vi "02 HEWH Heat Up Test SM1.vi"(0 "Equipment":T6={"MW100"="COM3", "AG34970"="MW100", "WT210"="A-34972A"}, 5 "Degree Setting":dbl=58.0, 7 "Flow rate setting":dbl=3.0, 11 "Error In":errorcluster) -> (15 "Error Out":errorcluster)   [LabVIEW 2014]
uses:
  <vilib>/Utility/file.llb/Write To Spreadsheet File (string).vi
  Type Definitions/Use Modes.ctl
  Type Definitions/HEWH_Mode.ctl
  Type Definitions/ValveBankPositions.ctl
  Type Definitions/Intellfaucet Mode.ctl
  <vilib>/Analysis/NI_AALBase.lvlib
  <vilib>/Analysis/baseanly.llb/Mean (DBL).vi
  Type Definitions/EquipReferences.ctl
  Type Definitions/Heating Modes.ctl
  Type Definitions/HEWH Tank Indicator.ctl
  Type Definitions/PowerElements.ctl
  Type Definitions/TestedFlowratesScenarios.ctl
panel:
  in  "Test Condition":T1=enum."Global, Tank"
  out "Label Array":string[](array[string])
  out "Use Agilent?":bool
  out "Voltage":dbl=240.0
  out "COM Port":refnum<visa-resource-name>
  out "Serial Data In":string
  out "LAN IP Address":string="192.168.25.3"
  out "Computer Name":string
  out "Ver.":string
  out "POWER":T2
  out "Tank Display":T3 {"TC6" format="%.2g"; "TIN" format="%.2g"; "TOUT" format="%.2g"; "Mean" format="%.2f"; "Std Dev" format="%.2f"; "TC5" format="%.2g"; "TC4" format="%.2g"; "TC3" format="%.2g"; "TC2" format="%.2g"; "TC1" format="%.2g"}
  in  "Function Tab":enum32{"Setup", "Test Status", "Charts"}(tab)
  out "MW100":refnum<visa-resource-name>
  out "FileName":path
  in  "Working File Directory":path=path "c:/data"
  out "Heating  Mode":T4=enum."Hybrid Heating"
  in  "DRM Mode":T5=3 items=["CRITICAL", "HIGH", "MEDIUM", "Normal"]
  out "Data Array":string[][](array[string])
  out "GEA2 HyperData":bool=TRUE
  in  "Expansion Tank?":bool=TRUE
  in  "Status Tab":T7(tab)=enum."Feedback 6"
  out "errorset mode":errorcluster
  out "Init Complete":bool
  out "Mode":T8=enum."HighDemand"
  out "Set Point":u8=140
  out "Heat Source Indicator":bool
  in  "SkipStabilize":bool
  out "Elapsed Time (secs)":dbl format="%.2f"
  in  "Stability Sample Delay(s)":dbl=120.0
  out "1.Delay Mins(30)":dbl
  in  "1.SkipDelay":bool
  out "Flowrate adj":dbl=3.0
  out "Downspout Flow Chart":dbl(graph)=3.8899999999999997
  in  "Time Delay(30)":dbl=30.0
  out "Temp adj":dbl=3.0
  out "Downspout Temp":dbl(graph)=3.8899999999999997
  out "2.Bottom Source Indicator":bool
  in  "2. Initial Draw":dbl=10.75
  out "3.WaitTime(10min)":dbl
  out "error 3":errorcluster
  out "3.Heat Source Indicator":bool
  in  "Wait Time(600s)":dbl=600.0
  out "4.Delay Remaining (300s)":dbl
  in  "Delay(300s)":dbl=300.0
  in  "4.Skip Delay":bool
  out "Downspout Flow Chart":dbl(graph)=3.8899999999999997
  out "Downspout Flow":dbl=3.8899999999999997
  out "Total Gal Out":dbl
  out "5.Top Source Indicator":bool
  in  "Eheat Gal Limit":dbl=40.0
  in  "Flow Adjust Time (3s)":dbl=1.5
  in  "K(0.1)":dbl=0.1
  in  "Total Gal Limit":dbl=200.0
  out "6.Bottom Source Indicator":bool
  in  "Delay eHeat Command (mS)":u32=15000
  in  "Skip Waiting for Bottom Source to turn off.":bool
  out "7.Heat Source Indicator":bool
  out "Mean Tank Temp":dbl
  in  "Min Ave Temp Limit":dbl=120.0
  in  "8.Skip Waiting":bool
  out "Seconds to Completion":dbl
  in  "8.Delay(1800s)":dbl=1800.0
  out "LoggingStopped":bool=TRUE
  out "Test Data":string[][](array[string])
  in  "Graph Tab":enum32{"Temperature", "Power", "Gallons"}(tab)
  out "Ave Temp":dbl format="%0.2f"
  out "Local?":bool
  # "Select the Modes for the test.  This will need to be\nset up on the water heater."
  # "Wait for stabilization.  Checks heat sources every second.  \nIf the heat sources are both off, the water heater is stabilized. \nFor StdElect. Looks at the heating element.  For other heating\nmodes, looks at the RS232 feedback on fans and compressor."
  # "\"1.\tAfter unit has been stable for 30+/-5 minutes, Open valve,\n and draw 10.75 +/- .25 gallons of water at a rate of 3+/-.25 gpm.\""
  # "First, Allow the water temp and flow to stabilize in the downspout,\nthen switch to the tank."
  # "\"2.\tIf lower heat source energizes (Hybrid Mode/eHeat Mode = FAN ON\nfollow by Compressor, Standard Electric Mode = Lower Element ON) \nbefore 10.75 gallons, then continue drawing water until Upper element \nengages as shown in step 5 (skip to step 5).\""
  # "\"3.\tIf lower heat source does not energize during 10.75 gallon draw, then wait a maximum of 10 minutes to see if lower heat source will energize.  If it does, then\nallow the water heater to recover to set point.\""
  # "\"4.\tAllow unit to sit 5 to 10 minutes in stabilized conditions, then:\""
  # "Change delay value to skip ahead."
  # "\"5.\tOpen valve and draw water at 3+/-.25 gpm until the Upper Element \nenergizes.  Water draw must stop within 5 seconds after Upper Element \nenergizes.  NOTE: when running the unit in e-Heat mode, (no upper \nelement) draw 40+/-0.25 gallons of water.\""
  # "\"6.\tIn Hybrid Mode: when the Upper Element stops and \nswitches to Lower Element, switch the unit to eHeat Mode.  \nThis will switch the lower heating source to Compressor.\""
  # "Since there may be a significant delay \nfor the compressor to turn on, also check \nto make sure that the mean tank temp\nis above some limit."
  # "7.\tAllow water heater to stabilize this second time. \n(Recover water temperature back to set point)."
  # "8.\tAllow unit to sit a minimum of 30 minutes in stabilized conditions, then;"
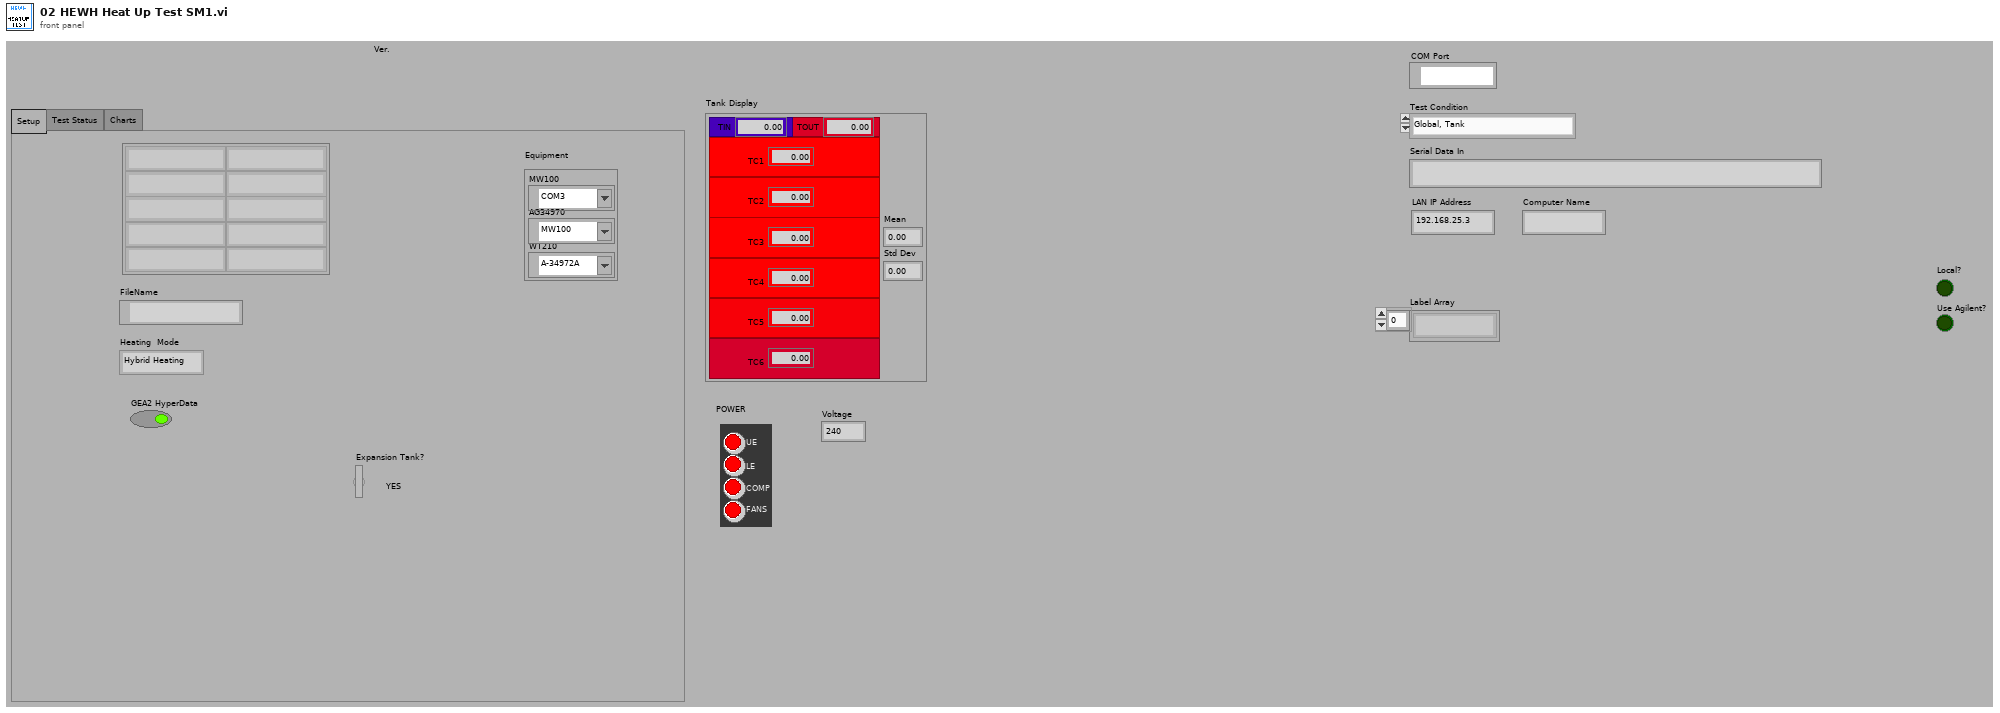
[diagram p1: front panel]
types:
  T1 = typedef "TestedFlowratesScenarios.ctl" = enum16{"DRK500,Station1", "DRK375,Lab", "SRK500,Station1,5GPM FR", "DRK375,STATION3,1/2\"HOSE", "DRK500,Station1,downspout", "DRK375,Station3,thruEcocute", "DRK375,Station3,purge", "Build2,2B,Purge", "Global, Purge", "Global, Tank", "DRK250"}
  T2 = typedef "PowerElements.ctl" = cluster{"UE":bool, "LE":bool, "COMP":bool, "FANS":bool}
  T3 = typedef "HEWH Tank Indicator.ctl" = cluster{"TC1-D":bool, "TC2-D":bool, "TC3-D":bool, "TC4-D":bool, "TC5-D":bool, "RTD_IN":bool, "RTDOUT":bool, "TC1":dbl, "TC2":dbl, "TC3":dbl, "TC4":dbl, "TC5":dbl, "TIN":dbl, "TOUT":dbl, "Std Dev":dbl, "Mean":dbl, "TC6-D":bool, "TC6":dbl}
  T4 = typedef "Heating Modes.ctl" = enum16{"Standard Electric", "Hybrid Heating", "E-Heat Mode"}
  T5 = typedef "Use Modes.ctl" = u16
  T6 = typedef "EquipReferences.ctl" = cluster{"MW100":refnum<visa-resource-name>, "AG34970":refnum<visa-resource-name>, "WT210":refnum<visa-resource-name>}
  T7 = enum32{"External Program Controls", "External Program Controls 2", "Program Controls", "Feedback", "Feedback 2", "Feedback 3", "Feedback 4", "Feedback 5", "Feedback 6", "Feedback 7", "Feedback 8", "Feedback 9", "Feedback 10"}
  T8 = typedef "HEWH_Mode.ctl" = enum16{"Hybrid", "StdElectric", "eHeat", "HighDemand", "Vacation"}
  T9 = typedef "Intellfaucet Mode.ctl" = enum16{"Adjust Temp", "Adjust Flow", "Start Flow", "Stop Flow"}
  T10 = typedef "ValveBankPositions.ctl" = enum16{"Heating", "Purge", "Resting", "Draw"}
  T11 = typedef "FileVersionInformation.ctl" = cluster{"FileVersion":string, "ProductName":string, "InternalName":string, "CompanyName":string, "LegalCopyright":string, "FileDescription":string}
  T12 = enum16{"Computation Start", "Computation stop", "Reset Computation", "Clear Computation"}[]
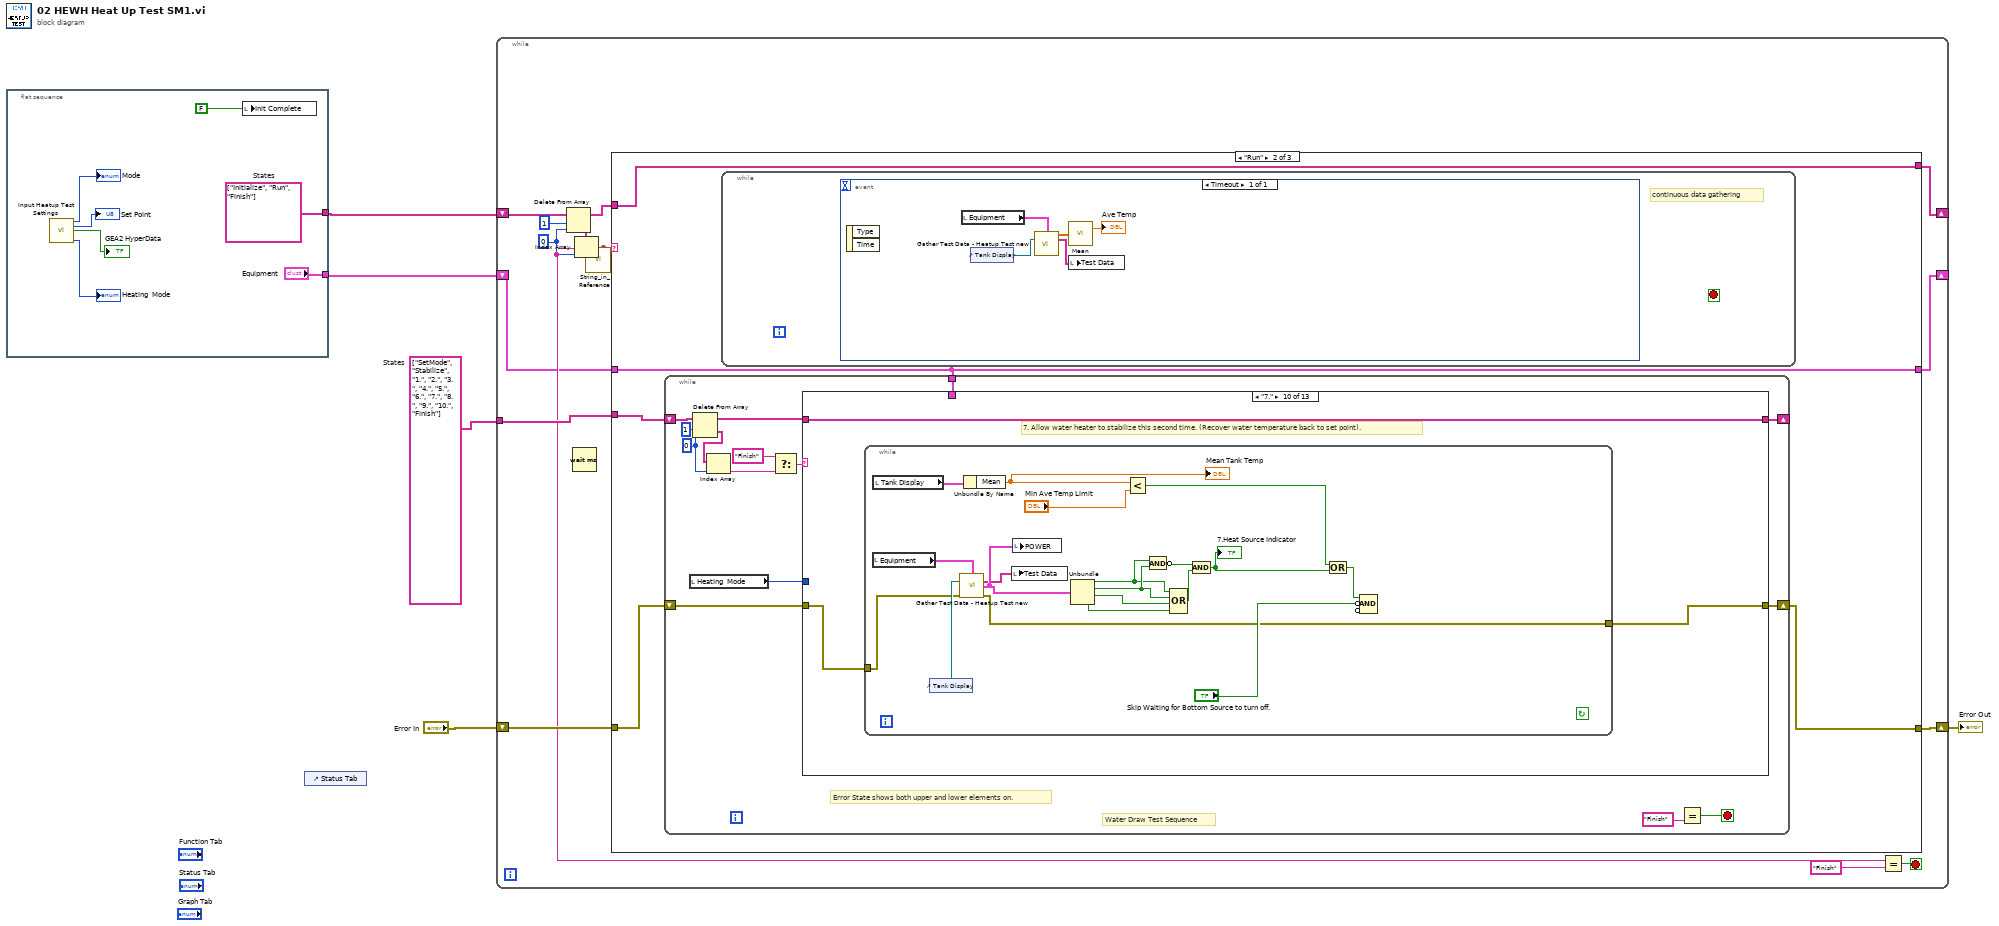
[diagram p0: block diagram]
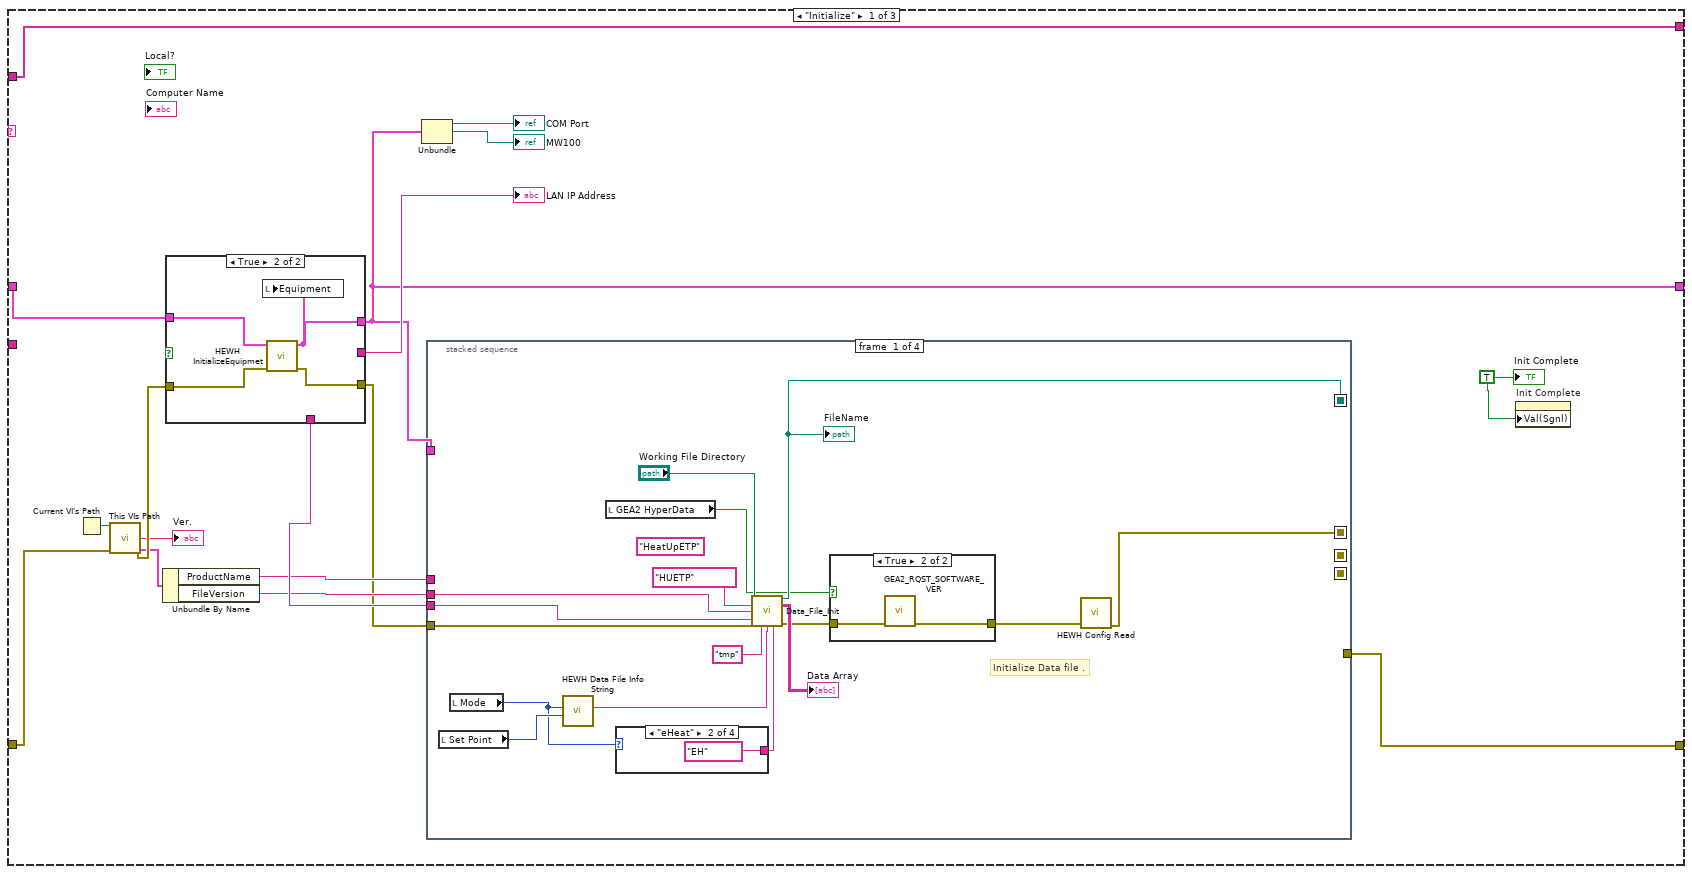
[diagram p2: hidden frame]
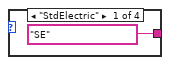
[diagram p4: hidden frame]
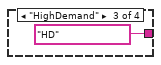
[diagram p5: hidden frame]
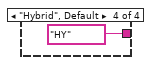
[diagram p6: hidden frame]
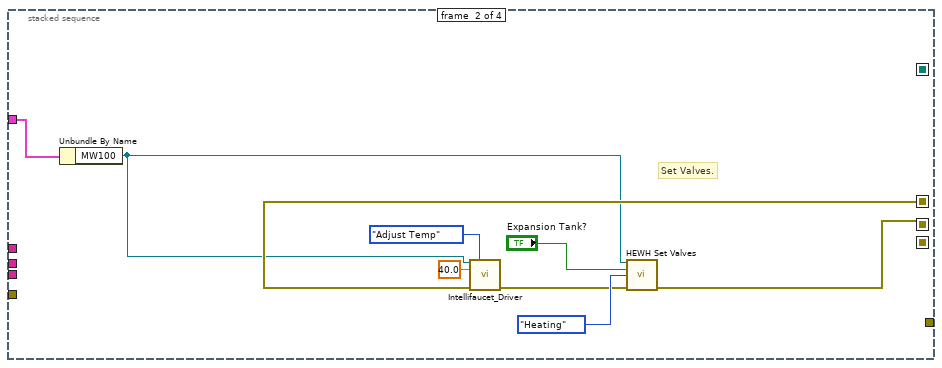
[diagram p7: hidden frame]
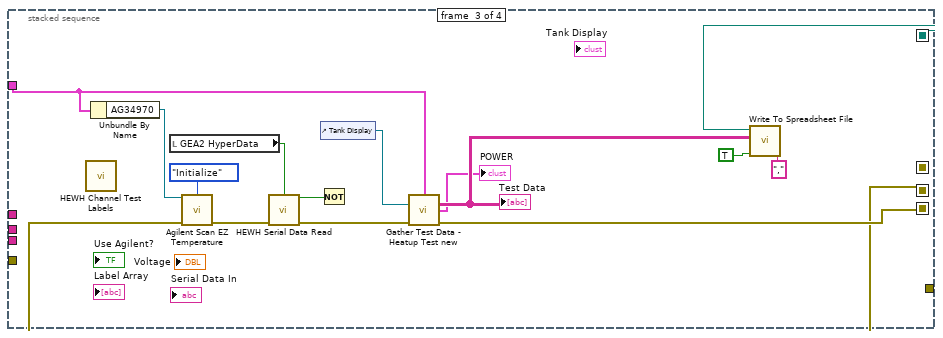
[diagram p8: hidden frame]
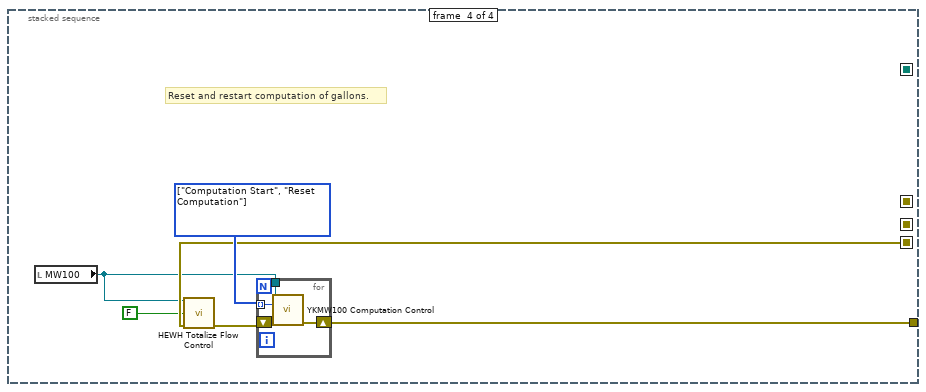
[diagram p9: hidden frame]
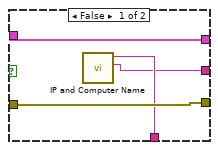
[diagram p10: hidden frame]
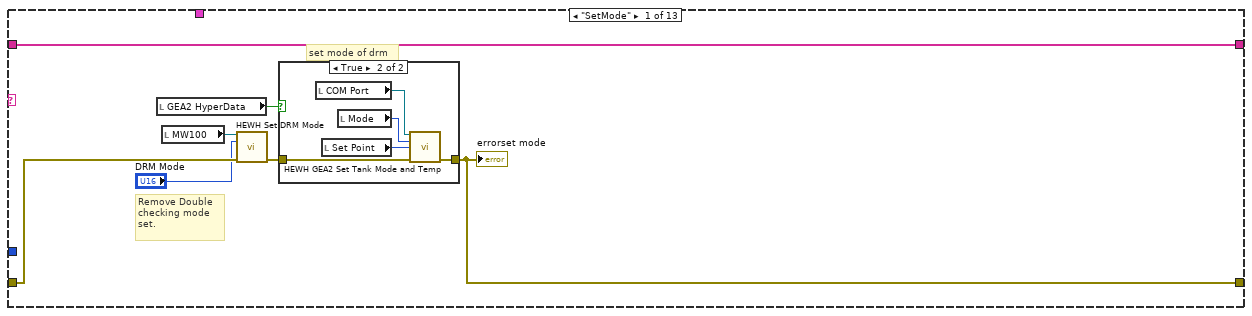
[diagram p11: hidden frame]
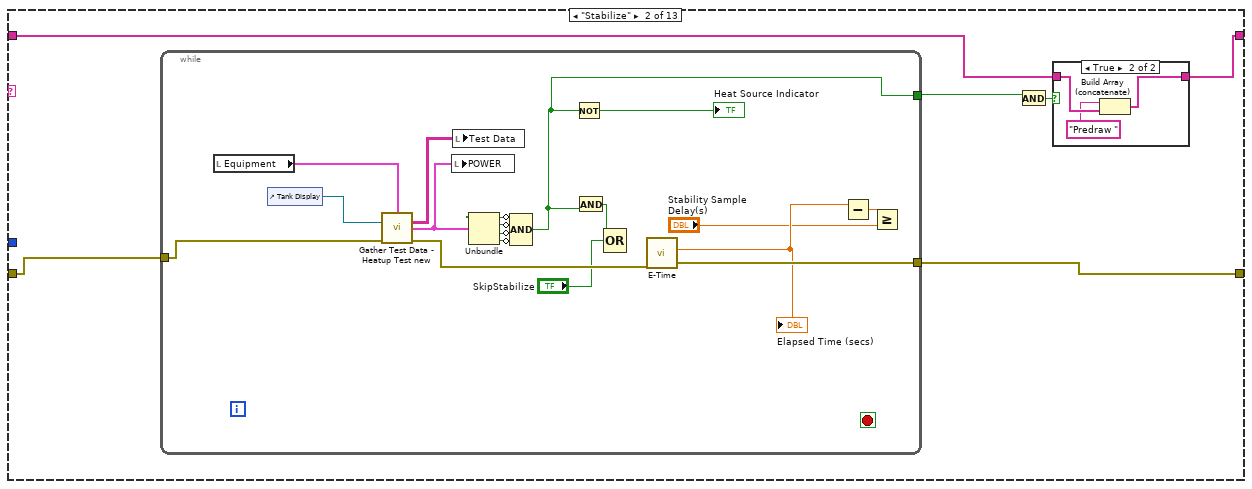
[diagram p13: hidden frame]
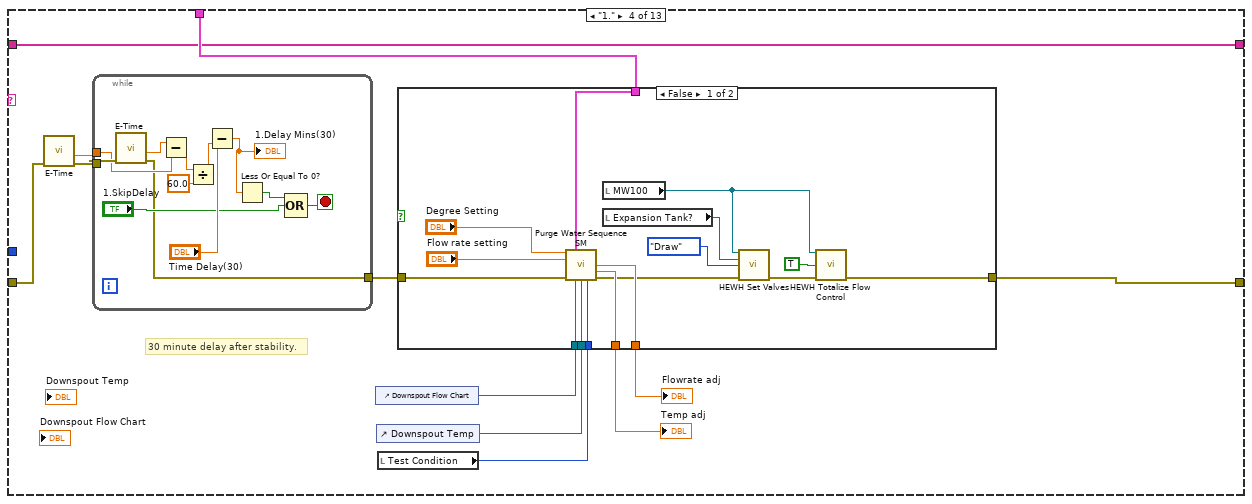
[diagram p16: hidden frame]
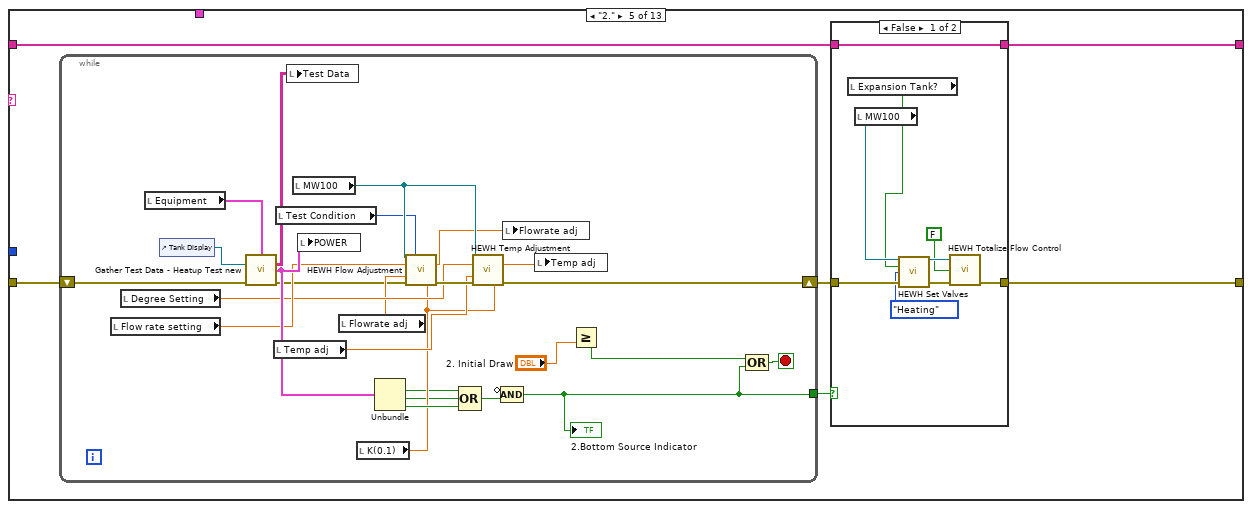
[diagram p18: hidden frame]
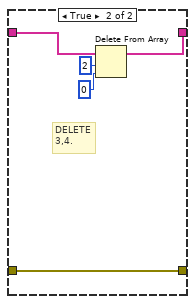
[diagram p19: hidden frame]
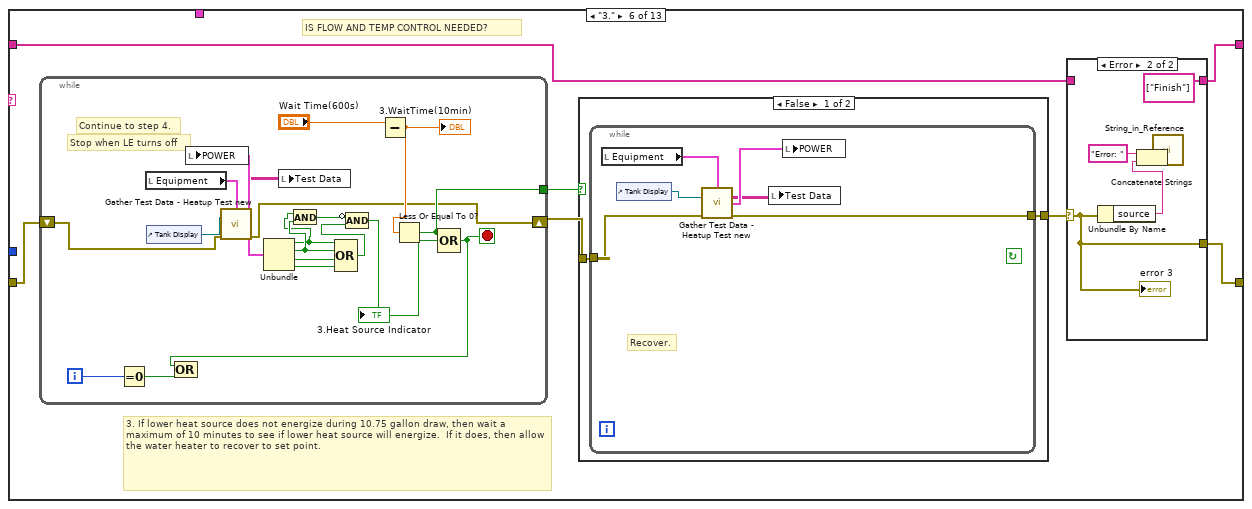
[diagram p20: hidden frame]
diagram:
  w3 = string[] ["SetMode", "Stabilize", "1.", "2.", "3.", "4.", "5.", "6.", "7.", "8.", "9.", "10.", "Finish"]  # States
  n1 = flat-sequence {
    tunnel: [w12] -> w5
    tunnel: ["Equipment"] -> w1
    frame #0 {
      w12 = string[] ["Initialize", "Run", "Finish"]  # States
      n2 = call "Input Heatup Test Settings.vi"() -> ("GEA2 Set Mode Out"=→"Mode":T8, "Set PointOut"=→"Set Point":u8, "GEA2 HyperData Out"=→"GEA2 HyperData":bool, "Heating  Mode Out"=→"Heating  Mode":T4)  [unwired: 11 in, 1 out]
      n3 = local write "Init Complete"(FALSE ("Init Complete")) -> ()
    }
  }
  n4 = control-ref of="Status Tab"() -> ()  [unwired: 1 out]
  n5 = while {
    shift-right: [w22] -> _
    shift-left: w5 -> [w26]
    shift-right: [w20] -> w4
    shift-left: "Error In" -> [w19]
    shift-right: [w16] -> _
    shift-left: w1 -> [w13]
    tunnel: w3 -> [w15]
    stop <- w18 stop-if-true
    w23 = 0 ("index")
    n6 = Delete From Array(array=w26, length=1, index=w23) -> (deleted portion=w24:string[], array with subset deleted=w21:string[])
    n7 = Wait (ms)() -> ()  [unwired: 1 in, 1 out]
    n8 = Index Array(array=w24, index=w23) -> (element=w14:string)
    n9 = call "String_in_Reference.vi"("String"=w14) -> ()  [unwired: 18 in, 1 out]
    n10 = case shown="\"Run\"" w14 {
      tunnel: [w41 w110 w463] -> w22
      tunnel: w21 -> [w41 w110 w463]
      tunnel: [w42 w109 w462] -> w20
      tunnel: w19 -> [w28 w112 w462]
      tunnel: w13 -> [w43 w111 w465]
      tunnel: [w34 w111 w465] -> w16
      tunnel: w15 -> [_ w113 _]
      frame "Initialize" {
        w27 = TRUE ("Init Complete")
        n11 = Current VI's Path() -> (path=w40:path)
        n12 = call "This VIs Path.vi"("path"=w40, "error in (no error)"=w28) -> ("File Version Info"=→"Ver.":string, "FileVersionInfo Out"=w32:T11, "error out"=w39:errorcluster)  [unwired: 9 in, 2 out]
        n13 = Unbundle By Name(w32) -> ("ProductName"=w31:string, "FileVersion"=w30:string)
        n14 = case shown="True" {
          selector: _ -> [_ _]
          tunnel: w39 -> [w104 w108]
          tunnel: w43 -> [w103 w105]
          tunnel: [w103 w106] -> w34
          tunnel: [w104 w107] -> w29
          tunnel: [w102 _] -> w33
          tunnel: [w101 _] -> w36
          frame False {
            n15 = call "IP and Computer Name.vi"() -> ("IP Address"=w101:string, "Computer Name"=w102:string)  [unwired: 10 in]
          }
          frame True {
            n16 = call "HEWH InitializeEquipmet.vi"("Error In"=w108, "Equipment"=w105) -> ("Error Out"=w107:errorcluster, "Equipment Out"=w106:T6)  [unwired: 8 in]
            n17 = local write "Equipment"(w106) -> ()
          }
        }
        "LAN IP Address" <- w36
        n18 = Unbundle(w34) -> ("MW100"=→"COM Port":refnum<visa-resource-name>, "AG34970"=→"MW100":refnum<visa-resource-name>)  [unwired: 1 out]
        n19 = stacked-sequence {
          seq-local: [_ w75 _ _] -> [_ _ w87 _]
          seq-local: [w51 _ _ _] -> [_ w70 _ _]
          seq-local: [_ _ w89 _] -> [_ _ _ w94]
          seq-local: [w48 _ _ _] -> [_ _ w88 _]
          tunnel: [_ _ _ w95] -> w42
          tunnel: w33 -> [w59 _ _ _]
          tunnel: w29 -> [w58 _ _ _]
          tunnel: w34 -> [_ w74 w90 _]
          tunnel: w31 -> [_ _ _ _]
          tunnel: w30 -> [w55 _ _ _]
          frame #0 {
            (unwired) "HeatUpETP" ("Test_Type In:")
            # "Initialize Data file ."
            n20 = local read "Set Point"() -> (w53:u8)
            n21 = local read "Mode"() -> (w47:T8)
            n22 = call "HEWH Data File Info String.vi"("Set PointOut"=w53, "GEA2 Set Mode"=w47) -> ("Info string"=w52:string)  [unwired: 9 in]
            n23 = local read "GEA2 HyperData"() -> (w44:bool)
            n24 = case shown="\"eHeat\"" w47 {
              tunnel: ["SE" ("Mode:") "EH" ("Mode:") "HD" ("Mode:") "HY" ("Mode:")] -> w46
              frame "StdElectric" {
              }
              frame "eHeat" {
              }
              frame "HighDemand" {
              }
              frame "Hybrid", Default {
              }
            }
            n25 = call "Data_File_Init.vi"("Data File Directory"="Working File Directory", "Test_Name In:"="HUETP", "Version In:"=w55, "Computer Name In:"=w59, "error in (no error)"=w58, "File Extension:"="tmp", "Ambient Temp / RH:"=w52, "Mode:"=w46) -> ("FileName"=w48:path, "Data Array"=→"Data Array":string[][], "error out"=w50:errorcluster)  [unwired: 5 in]
            "FileName" <- w48
            n26 = case shown="True" w44 {
              tunnel: w50 -> [w60 w62]
              tunnel: [w60 w61] -> w49
              frame False {
              }
              frame True {
                n27 = call "GEA2_RQST_SOFTWARE_VER.vi"("Error In"=w62) -> ("Error Out"=w61:errorcluster)  [unwired: 11 in, 3 out]
              }
            }
            n28 = call "HEWH Config Read.vi"("error in (no error)"=w49) -> ("error out"=w51:errorcluster)  [unwired: 13 in, 1 out]
          }
          frame #1 {
            # "Set Valves."
            n29 = Unbundle By Name(w74) -> ("MW100"=w69:refnum<visa-resource-name>)
            n30 = call "Intellifaucet_Driver.vi"("VISA session"=w69, "Mode"=Intellfaucet_Mode."Adjust Temp", "Temperature(F)"=40.0, "Error In"=w70) -> ("Error Out"=w71:errorcluster)  [unwired: 10 in, 1 out]
            n31 = call "HEWH Set Valves.vi"("VISA session"=w69, "Pressurize Tank?"="Expansion Tank?", "Valve Bank Setting"=ValveBankPositions."Heating", "Error In"=w71) -> ("Error Out"=w75:errorcluster)  [unwired: 10 in, 1 out]
          }
          frame #2 {
            n32 = call "HEWH Channel Test Labels.vi"() -> ()  [unwired: 13 in, 3 out]
            n33 = Unbundle By Name(w90) -> ("AG34970"=w84:refnum<visa-resource-name>)
            n34 = local read "GEA2 HyperData"() -> (w78:bool)
            n35 = call "Agilent Scan EZ Temperature.vi"("VISA Resource Name"=w84, "Control"=enum16{"Initialize", "Read", "Experiment"}."Initialize", "error in (no error)"=w87) -> ("error out"=w85:errorcluster)  [unwired: 9 in, 3 out]
            n36 = call "HEWH Serial Data Read.vi"("GEA2 HyperData"=w78, "error in (no error)"=w85) -> ("Serial Read OK"=w77:bool, "error out"=w76:errorcluster)  [unwired: 10 in, 2 out]
            n37 = Not(x=w77) -> ()  [unwired: 1 out]
            n38 = control-ref of="Tank Display"() -> (w81:refnum<vi>)
            n39 = call "Gather Test Data - Heatup Test new.vi"("Equipment"=w90, "Tank Display Ref"=w81, "error in (no error)"=w76) -> ("Output Data"=w80:string[][], "POWER"=→"POWER":T2, "error out"=w89:errorcluster)  [unwired: 8 in, 2 out]
            "Test Data" <- w80
            n40 = call-poly <vilib>:"Write To Spreadsheet File.vi"("delimiter (\\t)"="," ("delimiter (\\t)"), "append to file? (new file:F)"=TRUE, "2D data"=w80, "file path (dialog if empty)"=w88) -> ()  [unwired: 4 in, 1 out]
          }
          frame #3 {
            w96 = T12 [enum."Computation Start", enum."Reset Computation"] items=["Computation Start", "Computation stop", "Reset Computation", "Clear Computation"]
            # "Reset and restart computation of gallons."
            n41 = local read "MW100"() -> (w91:refnum<visa-resource-name>)
            n42 = call "HEWH Totalize Flow Control.vi"("VISA session"=w91, "Totalize Flow"=FALSE, "error in (no error)"=w94) -> ("error out"=w93:errorcluster)  [unwired: 11 in, 1 out]
            n43 = for {
              tunnel: w96 -> [w98] mode=indexing
              shift-right: [w99] -> w95
              shift-left: w93 -> [w100]
              tunnel: w91 -> [w97]
              n44 = call "YKMW100 Computation Control.vi"("VISA session"=w97, "Mode"=w98, "error in (no error)"=w100) -> ("error out"=w99:errorcluster)  [unwired: 11 in, 1 out]
            }
          }
        }
        n45 = property on="Init Complete" class="Bool (strict)"("Val(Sgnl)"=w27) -> ()  [unwired: 2 in, 2 out]
        "Init Complete" <- w27
      }
      frame "Run" {
        n46 = while {
          shift-right: [w124] -> _
          shift-left: w113 -> [w125]
          tunnel: w111 -> [w121]
          shift-right: [w116] -> w109
          shift-left: w112 -> [w114]
          stop <- w120 stop-if-true
          w126 = 0 ("index")
          # "Error State shows both upper and lower elements on."
          # "Water Draw Test Sequence"
          n47 = local read "Heating  Mode"() -> (w115:T4)
          n48 = Delete From Array(array=w125, length=1, index=w126) -> (deleted portion=w127:string[], array with subset deleted=w123:string[])
          n49 = Index Array(array=w127, index=w126) -> (element=w119:string)
          n50 = Select(t="Finish", f=w119) -> (s? t:f=w117:string)  [unwired: 1 in]
          n51 = case shown="\"7.\"" w117 {
            tunnel: w114 -> [w135 w142 _ w174 w213 w256 w298 w321 w364 w410 w434 w448 w450]
            tunnel: [w129 w147 _ w170 w211 w262 w300 w327 w362 w409 w433 w447 w451] -> w116
            tunnel: [w130 w146 _ w171 w212 w261 w301 w328 w361 w408 w431 w449 w453] -> w124
            tunnel: w123 -> [w130 w145 _ w171 w214 w260 w301 w328 w361 w408 w431 w449 w453]
            tunnel: w121 -> [_ _ _ w181 _ _ _ _ _ _ _ _ _]
            tunnel: w115 -> [_ _ _ _ _ _ _ w329 w363 _ _ _ _]
            frame "SetMode" {
              # "set mode of drm"
              # "Remove Double\nchecking mode \nset."
              n52 = local read "GEA2 HyperData"() -> (w131:bool)
              n53 = local read "MW100"() -> (w132:refnum<visa-resource-name>)
              n54 = call "HEWH Set DRM Mode.vi"("MW100"=w132, "Mode"="DRM Mode", "error in (no error)"=w135) -> ("error out"=w133:errorcluster)  [unwired: 12 in]
              n55 = case shown="True" w131 {
                tunnel: w133 -> [w136 w137]
                tunnel: [w136 w138] -> w129
                frame False {
                }
                frame True {
                  n56 = local read "COM Port"() -> (w139:refnum<visa-resource-name>)
                  n57 = local read "Set Point"() -> (w140:u8)
                  n58 = local read "Mode"() -> (w141:T8)
                  n59 = call "HEWH GEA2 Set Tank Mode and Temp.vi"("ComPort"=w139, "Mode"=w141, "Set Point"=w140, "Error In"=w137) -> ("Error Out"=w138:errorcluster)  [unwired: 9 in, 2 out]
                }
              }
              "errorset mode" <- w129
            }
            frame "Stabilize" {
              n60 = while {
                tunnel: w142 -> [w152]
                tunnel: [w169] -> w147
                tunnel: [w154] -> w144
                stop <- _ stop-if-true
                n61 = local read "Equipment"() -> (w165:T6)
                n62 = control-ref of="Tank Display"() -> (w164:refnum<vi>)
                n63 = call "Gather Test Data - Heatup Test new.vi"("Equipment"=w165, "Tank Display Ref"=w164, "error in (no error)"=w152) -> ("Output Data"=w161:string[][], "POWER"=w163:T2, "error out"=w162:errorcluster)  [unwired: 8 in, 2 out]
                n64 = local write "POWER"(w163) -> ()
                n65 = local write "Test Data"(w161) -> ()
                n66 = Unbundle(w163) -> ("UE"=w166:bool, "LE"=w167:bool, "COMP"=w168:bool, "FANS"=w160:bool)
                n67 = Compound Arithmetic op=AND(invert w166, invert w167, invert w168, invert w160) -> (w154:bool)
                n68 = Not(x=w154) -> (.not. x?=→"Heat Source Indicator":bool)
                n69 = And(y=w154) -> (x .and. y?=w159:bool)  [unwired: 1 in]
                n70 = Compound Arithmetic op=OR(w159, "SkipStabilize") -> ()  [unwired: 1 in, 1 out]
                n71 = call "E-Time.vi"("error in (no error)"=w162) -> ("error out"=w169:errorcluster, "Elapsed Time (sec)"=w157:dbl)  [unwired: 8 in, 1 out]
                "Elapsed Time (secs)" <- w157
                n72 = Subtract(x=w157) -> (x-y=w156:dbl)  [unwired: 1 in]
                n73 = Greater Or Equal?(x=w156, y="Stability Sample Delay(s)") -> ()  [unwired: 1 out]
              }
              n74 = And(x=w144) -> (x .and. y?=w143:bool)  [unwired: 1 in]
              n75 = case shown="True" w143 {
                tunnel: [w148 w151] -> w146
                tunnel: w145 -> [w148 w150]
                frame False {
                }
                frame True {
                  n76 = Build Array (concatenate)("Predraw " ("string"), w150) -> (w151:string[])
                }
              }
            }
            frame "Predraw" {
            }
            frame "1." {
              # "30 minute delay after stability."
              n77 = call "E-Time.vi"("error in (no error)"=w174) -> ("error out"=w173:errorcluster, "Elapsed Time (sec)"=w172:dbl)  [unwired: 8 in, 1 out]
              n78 = while {
                tunnel: [w199] -> w178
                tunnel: w173 -> [w207]
                tunnel: w172 -> [w200]
                stop <- w208 stop-if-true
                n79 = call "E-Time.vi"("error in (no error)"=w207) -> ("error out"=w199:errorcluster, "Elapsed Time (sec)"=w201:dbl)  [unwired: 8 in, 1 out]
                n80 = Subtract(x=w201, y=w200) -> (x-y=w202:dbl)
                n81 = Divide(x=w202, y=60.0) -> (x/y=w205:dbl)
                n82 = Subtract(x="Time Delay(30)", y=w205) -> (x-y=w204:dbl)
                "1.Delay Mins(30)" <- w204
                n83 = Less Or Equal To 0?(x=w204) -> (x <= 0?=w209:bool)
                n84 = Compound Arithmetic op=OR(w209, "1.SkipDelay") -> (w208:bool)  [unwired: 1 in]
              }
              n85 = control-ref of="Downspout Flow Chart"() -> (w179:refnum<vi>)
              n86 = control-ref of="Downspout Temp"() -> (w175:refnum<vi>)
              n87 = local read "Test Condition"() -> (w177:T1)
              n88 = case shown="False" {
                selector: _ -> [_ _]
                tunnel: w181 -> [w195 _]
                tunnel: [w186 w198] -> w170
                tunnel: [w194 _] -> w180
                tunnel: w179 -> [w193 _]
                tunnel: w178 -> [w182 w198]
                tunnel: w177 -> [w192 _]
                tunnel: [w191 _] -> w176
                tunnel: w175 -> [w190 _]
                frame False {
                  n89 = call "Purge Water Sequence SM.vi"("Degree Setting"="Degree Setting", "Equipment"=w195, "Flow rate setting"="Flow rate setting", "Error In"=w182, "Flow Chart Ref"=w193, "Temp Chart Ref"=w190, "Test Condition"=w192) -> ("Flow rate setting out"=w194:dbl, "Temp Setting Out"=w191:dbl, "Error Out"=w183:errorcluster)  [unwired: 3 in, 3 out]
                  n90 = local read "MW100"() -> (w185:refnum<visa-resource-name>)
                  n91 = local read "Expansion Tank?"() -> (w188:bool)
                  n92 = call "HEWH Set Valves.vi"("VISA session"=w185, "Pressurize Tank?"=w188, "Valve Bank Setting"=ValveBankPositions."Draw", "Error In"=w183) -> ("Error Out"=w187:errorcluster)  [unwired: 10 in, 1 out]
                  n93 = call "HEWH Totalize Flow Control.vi"("VISA session"=w185, "Totalize Flow"=TRUE, "error in (no error)"=w187) -> ("error out"=w186:errorcluster)  [unwired: 11 in, 1 out]
                }
                frame True {
                }
              }
              "Flowrate adj" <- w180
              "Temp adj" <- w176
            }
            frame "2." {
              n94 = while {
                tunnel: [w234] -> w215
                shift-right: [w246] -> w216
                shift-left: w213 -> [w253]
                stop <- w249 stop-if-true
                n95 = local read "Flow rate setting"() -> (w242:dbl)
                n96 = local read "Degree Setting"() -> (w241:dbl)
                n97 = local read "Equipment"() -> (w252:T6)
                n98 = control-ref of="Tank Display"() -> (w251:refnum<vi>)
                n99 = call "Gather Test Data - Heatup Test new.vi"("Equipment"=w252, "Tank Display Ref"=w251, "error in (no error)"=w253) -> ("Output Data"=w243:string[][], "POWER"=w254:T2, "error out"=w231:errorcluster)  [unwired: 8 in, 2 out]
                n100 = local read "Temp adj"() -> (w237:dbl)
                n101 = local read "Test Condition"() -> (w244:T1)
                n102 = local write "Test Data"(w243) -> ()
                n103 = local read "MW100"() -> (w245:refnum<visa-resource-name>)
                n104 = local write "POWER"(w254) -> ()
                n105 = local read "Flowrate adj"() -> (w238:dbl)
                n106 = local read "K(0.1)"() -> (w236:dbl)
                n107 = Unbundle(w254) -> ("LE"=w232:bool, "COMP"=w235:bool, "FANS"=w248:bool)  [unwired: 1 out]
                n108 = call "HEWH Flow Adjustment.vi"("VISA session"=w245, "Configuration"=w244, "GPM Target(3)"=w242, "New GPM Reading \nfrom last adjustment"=w238, "Error In"=w231, "K(0.2)"=w236) -> ("Flow rate setting Out"=w239:dbl, "Error Out"=w247:errorcluster)  [unwired: 6 in, 2 out]
                n109 = Compound Arithmetic op=OR(w232, w235, w248) -> (w233:bool)
                n110 = call "HEWH Temp Adjustment.vi"("VISA session"=w245, "Degrees Target"=w241, "New Temp Reading \nfrom last adjustment"=w237, "Error In"=w247, "K(0.1)"=w236) -> ("Degree setting Out"=w240:dbl, "Error Out"=w246:errorcluster)  [unwired: 8 in, 1 out]
                n111 = Compound Arithmetic op=AND(w233) -> (w234:bool)  [unwired: 1 in]
                "2.Bottom Source Indicator" <- w234
                n112 = local write "Flowrate adj"(w239) -> ()
                n113 = local write "Temp adj"(w240) -> ()
                n114 = Greater Or Equal?(y="2. Initial Draw") -> (x >= y?=w250:bool)  [unwired: 1 in]
                n115 = Compound Arithmetic op=OR(w250, w234) -> (w249:bool)
              }
              n116 = case shown="False" w215 {
                tunnel: [w225 w230] -> w211
                tunnel: w216 -> [w223 w230]
                tunnel: [w224 w229] -> w212
                tunnel: w214 -> [w224 w228]
                frame False {
                  n117 = local read "Expansion Tank?"() -> (w219:bool)
                  n118 = local read "MW100"() -> (w220:refnum<visa-resource-name>)
                  n119 = call "HEWH Set Valves.vi"("VISA session"=w220, "Pressurize Tank?"=w219, "Valve Bank Setting"=ValveBankPositions."Heating", "Error In"=w223) -> ("dup VISA session"=w221:refnum<visa-resource-name>, "Error Out"=w222:errorcluster)  [unwired: 10 in]
                  n120 = call "HEWH Totalize Flow Control.vi"("VISA session"=w221, "Totalize Flow"=FALSE, "error in (no error)"=w222) -> ("error out"=w225:errorcluster)  [unwired: 11 in, 1 out]
                }
                frame True {
                  # "DELETE\n3,4."
                  n121 = Delete From Array(array=w228, length=2, index=0) -> (array with subset deleted=w229:string[])  [unwired: 1 out]
                }
              }
            }
            frame "3." {
              # "IS FLOW AND TEMP CONTROL NEEDED?"
              # "3.\tIf lower heat source does not energize during 10.75 gallon draw, then wait a maximum of 10 minutes to see if lower heat source will energize.  If it does, then allow the water heater to recover to set point."
              n122 = while {
                tunnel: [w289] -> w259
                shift-right: [w272] -> w258
                shift-left: w256 -> [w285]
                i -> [w279]
                stop <- w281 stop-if-true
                # "Continue to step 4."
                # "Stop when LE turns off"
                n123 = Equal To 0?(x=w279) -> (x = 0?=w280:bool)
                n124 = local read "Equipment"() -> (w287:T6)
                n125 = control-ref of="Tank Display"() -> (w286:refnum<vi>)
                n126 = call "Gather Test Data - Heatup Test new.vi"("Equipment"=w287, "Tank Display Ref"=w286, "error in (no error)"=w285) -> ("Output Data"=w282:string[][], "POWER"=w284:T2, "error out"=w272:errorcluster)  [unwired: 8 in, 2 out]
                n127 = local write "POWER"(w284) -> ()
                n128 = Unbundle(w284) -> ("UE"=w273:bool, "LE"=w274:bool, "COMP"=w283:bool, "FANS"=w278:bool)
                n129 = local write "Test Data"(w282) -> ()
                n130 = And(x=w273, y=w274) -> (x .and. y?=w275:bool)
                n131 = Compound Arithmetic op=OR(w273, w274, w283, w278) -> (w276:bool)
                n132 = Compound Arithmetic op=AND(invert w275, w276) -> (w277:bool)
                "3.Heat Source Indicator" <- w277
                n133 = Subtract(x="Wait Time(600s)") -> (x-y=w288:dbl)  [unwired: 1 in]
                "3.WaitTime(10min)" <- w288
                n134 = Less Or Equal To 0?(x=w288) -> (x <= 0?=w289:bool)
                n135 = Compound Arithmetic op=OR(w289, w277) -> (w281:bool)  [unwired: 1 in]
                n136 = Compound Arithmetic op=OR(w281, w280) -> ()  [unwired: 1 out]
              }
              n137 = case shown="False" w259 {
                tunnel: w258 -> [w264 _]
                tunnel: [w263 errorcluster {"status"=TRUE, "code"=7003, "source"="FAIL!. Heating did not come on in time."} ("error out")] -> w257
                frame False {
                  n138 = while {
                    tunnel: w264 -> [w267]
                    tunnel: [w266] -> w263
                    stop <- _ continue-if-true
                    # "Recover."
                    n139 = local read "Equipment"() -> (w268:T6)
                    n140 = control-ref of="Tank Display"() -> (w269:refnum<vi>)
                    n141 = call "Gather Test Data - Heatup Test new.vi"("Equipment"=w268, "Tank Display Ref"=w269, "error in (no error)"=w267) -> ("Output Data"=w265:string[][], "POWER"=w270:T2, "error out"=w266:errorcluster)  [unwired: 8 in, 2 out]
                    n142 = local write "Test Data"(w265) -> ()
                    n143 = local write "POWER"(w270) -> ()
                  }
                }
                frame True {
                }
              }
              n144 = case shown="Error" w257 {
                selector: w257 -> [w291 w293]
                tunnel: [w292 string[] ["Finish"] ("States")] -> w261
                tunnel: w260 -> [w292 _]
                tunnel: [w291 w293] -> w262
                frame No Error {
                }
                frame Error {
                  n145 = Unbundle By Name(w293) -> ("source"=w296:string)
                  n146 = Concatenate Strings("Error: " ("string"), w296) -> (w294:string)
                  n147 = call "String_in_Reference.vi"("String"=w294) -> ()  [unwired: 18 in, 1 out]
                  "error 3" <- w293
                }
              }
            }
            frame "4." {
              # "4.\tAllow unit to sit 5 to 10 minutes in stabilized conditions, then:"
              n148 = call "E-Time.vi"("error in (no error)"=w298) -> ("error out"=w302:errorcluster, "Elapsed Time (sec)"=w299:dbl)  [unwired: 8 in, 1 out]
              n149 = while {
                tunnel: w302 -> [w312]
                tunnel: [w310] -> w300
                tunnel: w299 -> [w304]
                stop <- w309 continue-if-true
                n150 = call "E-Time.vi"("error in (no error)"=w312) -> ("error out"=w310:errorcluster, "Elapsed Time (sec)"=w305:dbl)  [unwired: 8 in, 1 out]
                n151 = Subtract(x=w305, y=w304) -> (x-y=w303:dbl)
                n152 = Subtract(x="Delay(300s)", y=w303) -> (x-y=w311:dbl)
                "4.Delay Remaining (300s)" <- w311
                n153 = Greater Than 0?(x=w311) -> (x > 0?=w308:bool)
                n154 = Compound Arithmetic op=AND(w308, invert "4.Skip Delay") -> (w309:bool)  [unwired: 1 in]
              }
            }
            frame "5." {
              n155 = local read "MW100"() -> (w320:refnum<visa-resource-name>)
              n156 = call "Solenoid Bank.vi"("VISA session"=w320, "Drain Valve"=enum8{"OPEN", "CLOSE"}."CLOSE", "Output Valve"=enum8{"CLOSE", "OPEN"}."OPEN", "Input Valve"=enum8{"OPEN", "CLOSE"}."OPEN", "Error In"=w321) -> ("dup VISA session"=w319:refnum<visa-resource-name>, "Error Out"=w322:errorcluster)  [unwired: 9 in]
              n157 = call "HEWH Totalize Flow Control.vi"("VISA session"=w319, "Totalize Flow"=TRUE, "error in (no error)"=w322) -> ("error out"=w324:errorcluster)  [unwired: 11 in, 1 out]
              n158 = while {
                shift-right: [w343] -> w326
                shift-left: w324 -> [w346]
                tunnel: w329 -> [w353]
                tunnel: [w352] -> w325
                stop <- _ stop-if-true
                n159 = control-ref of="Tank Display"() -> (w348:refnum<vi>)
                n160 = local read "Flow rate setting"() -> (w337:dbl)
                n161 = local read "Degree Setting"() -> (w338:dbl)
                n162 = local read "Equipment"() -> (w349:T6)
                n163 = call "Gather Test Data - Heatup Test new.vi"("Equipment"=w349, "Tank Display Ref"=w348, "error in (no error)"=w346) -> ("Output Data"=w340:string[][], "POWER"=w345:T2, "error out"=w330:errorcluster)  [unwired: 8 in, 2 out]
                n164 = local write "Test Data"(w340) -> ()
                n165 = local read "MW100"() -> (w344:refnum<visa-resource-name>)
                n166 = local write "POWER"(w345) -> ()
                n167 = call "Array_Search_For_Num.vi"("N Rows of Data"=w340, "Title?"="Tc_down") -> ("number"=w339:dbl)  [unwired: 12 in, 1 out]
                n168 = call "Array_Search_For_Num.vi"("N Rows of Data"=w340, "Title?"="FLOW(GPM)") -> ("number"=w347:dbl)  [unwired: 12 in, 1 out]
                "Downspout Flow" <- w347
                "Downspout Flow Chart" <- w347
                n169 = call "Array_Search_For_Num.vi"("N Rows of Data"=w340, "Title?"="GALLONS") -> ("number"=w332:dbl)  [unwired: 12 in, 1 out]
                "Total Gal Out" <- w332
                n170 = call "HEWH Flow Adjustment.vi"("VISA session"=w344, "Configuration"="Test Condition", "GPM Target(3)"=w337, "GPM reading"=w347, "Error In"=w330, "K(0.2)"="K(0.1)") -> ("VISA session out"=w336:refnum<visa-resource-name>, "Error Out"=w342:errorcluster)  [unwired: 6 in, 2 out]
                n171 = call "HEWH Temp Adjustment.vi"("VISA session"=w336, "Degrees Target"=w338, "Degrees reading"=w339, "Error In"=w342, "K(0.1)"="K(0.1)") -> ("Error Out"=w343:errorcluster)  [unwired: 8 in, 2 out]
                n172 = case shown="Default" w353 {
                  tunnel: w332 -> [w355 _]
                  tunnel: [w354 w358] -> w352
                  tunnel: w345 -> [_ w359]
                  frame "E-Heat Mode" {
                    n173 = Greater Or Equal?(x=w355, y="Eheat Gal Limit") -> (x >= y?=w354:bool)
                  }
                  frame Default {
                    n174 = Unbundle(w359) -> ("UE"=w360:bool, "LE"=w357:bool)  [unwired: 2 out]
                    n175 = Compound Arithmetic op=AND(w360, invert w357) -> (w358:bool)
                  }
                }
                n176 = Greater Or Equal?(x=w332, y="Total Gal Limit") -> (x >= y?=w331:bool)
                n177 = Compound Arithmetic op=OR(w331, w352) -> ()  [unwired: 1 out]
              }
              "5.Top Source Indicator" <- w325
              n178 = local read "Expansion Tank?"() -> (w314:bool)
              n179 = local read "MW100"() -> (w315:refnum<visa-resource-name>)
              n180 = call "HEWH Set Valves.vi"("VISA session"=w315, "Pressurize Tank?"=w314, "Valve Bank Setting"=ValveBankPositions."Heating", "Error In"=w326) -> ("Error Out"=w327:errorcluster)  [unwired: 10 in, 1 out]
            }
            frame "6." {
              # "6.\tIn Hybrid Mode: when the Upper Element stops and switches to Lower Element, switch the unit to eHeat Mode.  This will switch the lower heating source to Compressor."
              n181 = case shown="Default" w363 {
                tunnel: w364 -> [w365 w366]
                tunnel: [w365 w367] -> w362
                frame Default {
                }
                frame "Hybrid Heating" {
                  n182 = while {
                    shift-right: [w380] -> w367
                    shift-left: w366 -> [w368]
                    stop <- _ stop-if-true
                    # "Sample the beginning and end."
                    n183 = local read "Equipment"() -> (w378:T6)
                    n184 = control-ref of="Tank Display"() -> (w377:refnum<vi>)
                    n185 = call "Gather Test Data - Heatup Test new.vi"("Equipment"=w378, "Tank Display Ref"=w377, "error in (no error)"=w368) -> ("Output Data"=w376:string[][], "POWER"=w379:T2, "error out"=w375:errorcluster)  [unwired: 8 in, 2 out]
                    n186 = local write "Test Data"(w376) -> ()
                    n187 = local write "POWER"(w379) -> ()
                    n188 = local read "GEA2 HyperData"() -> (w374:bool)
                    n189 = Unbundle(w379) -> ("UE"=w371:bool, "LE"=w372:bool, "COMP"=w369:bool)  [unwired: 1 out]
                    n190 = Compound Arithmetic op=AND(invert w371, w372) -> (w370:bool)
                    n191 = Or(x=w370, y=w369) -> (x .or. y?=w373:bool)
                    "6.Bottom Source Indicator" <- w373
                    n192 = case shown="True" w374 {
                      tunnel: [w383 w395] -> w380
                      tunnel: w373 -> [w382 w394]
                      tunnel: w375 -> [w381 w393]
                      frame False {
                        n193 = case shown="True" w382 {
                          tunnel: [FALSE ("true") TRUE ("true")] -> _
                          tunnel: w381 -> [w385 w391]
                          tunnel: [w385 w386] -> w383
                          frame False {
                          }
                          frame True {
                            w389 = T5 2 items=["CRITICAL", "HIGH", "MEDIUM", "Normal"] ("Mode")
                            n194 = local read "MW100"() -> (w390:refnum<visa-resource-name>)
                            n195 = call "HEWH Set DRM Mode.vi"("MW100"=w390, "Mode"=w389, "error in (no error)"=w391) -> ("error out"=w388:errorcluster)  [unwired: 12 in]
                            n196 = call "Log String to Spreadsheet.vi"("String"="Set Mode to Medium", "error in (no error)"=w388) -> ("error out"=w386:errorcluster)  [unwired: 9 in]
                          }
                        }
                      }
                      frame True {
                        n197 = case shown="True" w394 {
                          tunnel: w393 -> [w396 w398]
                          tunnel: [w396 w397] -> w395
                          frame False {
                          }
                          frame True {
                            w406 = HEWH_Mode."eHeat" ("Mode")
                            n198 = local read "COM Port"() -> (w407:refnum<visa-resource-name>)
                            n199 = call "Delay mS.vi"("Error In"=w398, "milliseconds to wait"="Delay eHeat Command (mS)") -> ("Error Out"=w400:errorcluster)  [unwired: 13 in]
                            n200 = call "GEA2_CMD_UPDATE_MODE.vi"("ComPort"=w407, "Mode"=w406, "Error In"=w400) -> ("Error Out"=w401:errorcluster)  [unwired: 10 in, 2 out]
                            n201 = call "GEA2_RQST_STATUS_QUERY.vi"("ComPort"=w407, "Error In"=w401) -> ("Mode"=w405:T8, "Error Out"=w397:errorcluster)  [unwired: 8 in, 4 out]
                            n202 = Equal?(x=w406, y=w405) -> (x = y?=w402:bool)
                            n203 = Select(t="Set Mode to eHeat" ("String"), s=w402, f="Fail Set Mode to eHeat" ("String")) -> ()  [unwired: 1 out]
                          }
                        }
                      }
                    }
                  }
                }
              }
            }
            frame "7." {
              # "7.\tAllow water heater to stabilize this second time. (Recover water temperature back to set point)."
              n204 = while {
                tunnel: w410 -> [w424]
                tunnel: [w425] -> w409
                stop <- _ continue-if-true
                n205 = local read "Equipment"() -> (w427:T6)
                n206 = local read "Tank Display"() -> (w420:T3)
                n207 = control-ref of="Tank Display"() -> (w426:refnum<vi>)
                n208 = call "Gather Test Data - Heatup Test new.vi"("Equipment"=w427, "Tank Display Ref"=w426, "error in (no error)"=w424) -> ("Output Data"=w421:string[][], "POWER"=w428:T2, "error out"=w425:errorcluster)  [unwired: 8 in, 2 out]
                n209 = Unbundle By Name(w420) -> ("Mean"=w419:dbl)
                "Mean Tank Temp" <- w419
                n210 = local write "Test Data"(w421) -> ()
                n211 = local write "POWER"(w428) -> ()
                n212 = Unbundle(w428) -> ("UE"=w413:bool, "LE"=w414:bool, "COMP"=w423:bool, "FANS"=w422:bool)
                n213 = Less?(x=w419, y="Min Ave Temp Limit") -> (x < y?=w416:bool)
                n214 = Compound Arithmetic op=AND(w413, w414) -> (invert w411:bool)
                n215 = Compound Arithmetic op=OR(w413, w414, w423, w422) -> (w417:bool)
                n216 = And(x=w411, y=w417) -> (x .and. y?=w412:bool)
                "7.Heat Source Indicator" <- w412
                n217 = Or(x=w416, y=w412) -> (x .or. y?=w415:bool)
                n218 = Compound Arithmetic op=AND(w415, invert "Skip Waiting for Bottom Source to turn off.") -> ()  [unwired: 1 in, 1 out]
              }
            }
            frame "8." {
              n219 = call "E-Time.vi"("error in (no error)"=w434) -> ("error out"=w432:errorcluster, "Elapsed Time (sec)"=w430:dbl)  [unwired: 8 in, 1 out]
              n220 = while {
                shift-right: [w443] -> w433
                shift-left: w432 -> [w444]
                tunnel: w430 -> [w439]
                stop <- w437 continue-if-true
                # "8.\tAllow unit to sit a minimum of 30 minutes in stabilized conditions, then;"
                n221 = call "E-Time.vi"("error in (no error)"=w444) -> ("error out"=w443:errorcluster, "Elapsed Time (sec)"=w440:dbl)  [unwired: 8 in, 1 out]
                n222 = Subtract(x=w440, y=w439) -> (x-y=w438:dbl)
                n223 = Subtract(x="8.Delay(1800s)", y=w438) -> (x-y=w442:dbl)
                "Seconds to Completion" <- w442
                n224 = Greater Than 0?(x=w442) -> (x > 0?=w435:bool)
                n225 = Compound Arithmetic op=AND(w435, invert "8.Skip Waiting") -> (w437:bool)  [unwired: 1 in]
              }
            }
            frame "9." {
              w445 = T5 3 items=["CRITICAL", "HIGH", "MEDIUM", "Normal"] ("Mode")
              # "(Set DRM back to Normal)"
              # "9.\tStop Data Logger and HyperTerminal session."
              n226 = local read "MW100"() -> (w446:refnum<visa-resource-name>)
              n227 = call "HEWH Set DRM Mode.vi"("MW100"=w446, "Mode"=w445, "error in (no error)"=w448) -> ("error out"=w447:errorcluster)  [unwired: 12 in]
            }
            frame "Finish", Default {
              # "Stop Serail Data"
              # "Wait till logging loop completes"
              n228 = while {
                tunnel: [TRUE ("Stop Logging")] -> w452
                tunnel: [w454] -> w451
                tunnel: w450 -> [w454]
                stop <- _ stop-if-true
              }
              n229 = case shown="True" w452 {
                tunnel: w451 -> [_ _]
                frame False {
                }
                frame True {
                  "LoggingStopped" <- TRUE
                }
              }
            }
          }
          n230 = Equal?(y="Finish") -> (x = y?=w120:bool)  [unwired: 1 in]
        }
        n231 = while {
          stop <- _ stop-if-true
          # "continuous data gathering"
          n232 = event shown="[0] Timeout" {
            selector: _ -> [_]
            dyn-events: _ -> [_]
            timeout: _ -> [_]
            event Timeout {
              n233 = event-data() -> ()  [unwired: 1 in, 2 out]
              n234 = local read "Equipment"() -> (w461:T6)
              n235 = control-ref of="Tank Display"() -> (w460:refnum<vi>)
              n236 = call "Gather Test Data - Heatup Test new.vi"("Equipment"=w461, "Tank Display Ref"=w460) -> ("Tc Tree"=w458:dbl[], "Output Data"=w459:string[][])  [unwired: 9 in, 3 out]
              n237 = call-poly <vilib>:"Mean.vi"("X"=w458) -> ("mean"=→"Ave Temp":dbl)  [unwired: 1 out]
              n238 = local write "Test Data"(w459) -> ()
            }
          }
        }
      }
      frame "Finish", Default {
        n239 = property on="Init Complete" class="Bool (strict)"("Val(Sgnl)"=TRUE) -> ()  [unwired: 2 in, 2 out]
      }
    }
    n240 = Equal?(x=w14, y="Finish") -> (x = y?=w18:bool)
  }
  "Error Out" <- w4
